vi "ep_Inverse Curves Constants.vi"(9 "other curves index":i32, 10 "IEEE curve type":u16(ring) items=["IEEE moderately inverse", "IEEE very inverse", "IEEE extremely inverse"], 11 "IEC curve type":u16(ring) items=["IEC inverse", "IEC very inverse", "IEC extremely inverse"]) -> (0 "other curve parameters":T1={"operate time parameters"={"A [s]"=1.0, "B [s]"=1.0, "alpha"=1.0, "K2 [s]"=1.0, "K1 [s]"=1.0, "K3 [s]"=1.0}, "reset time parameters"={"tr [s]"=1.0, "alpha"=1.0}}, 1 "difference of 1/time":fxp<+/-,21,-17>, 2 "1/time":fxp<+/-,30,-10>, 3 "number of sections in each G/Gs step":u16=8, 4 "IEC parameters":T1={"operate time parameters"={"A [s]"=1.0, "B [s]"=1.0, "alpha"=1.0, "K2 [s]"=1.0, "K1 [s]"=1.0, "K3 [s]"=1.0}, "reset time parameters"={"tr [s]"=1.0, "alpha"=1.0}}, 6 "IEEE parameters":T1={"operate time parameters"={"A [s]"=1.0, "B [s]"=1.0, "alpha"=1.0, "K2 [s]"=1.0, "K1 [s]"=1.0, "K3 [s]"=1.0}, "reset time parameters"={"tr [s]"=1.0, "alpha"=1.0}})   [LabVIEW 2012, in "NI_EP_Protection.lvlib"]
uses:
  <vilib>/addons/Electrical Power/Protection/NI_EP_Protection.lvlib
  <vilib>/addons/Electrical Power/Protection/Inverse Time Delay/subVIs/ep_Curve Parameters.ctl
  <vilib>/addons/Electrical Power/Protection/Inverse Time Delay/subVIs/ep_Operate Time.ctl
  <vilib>/addons/Electrical Power/Protection/Inverse Time Delay/subVIs/ep_Reset Time.ctl
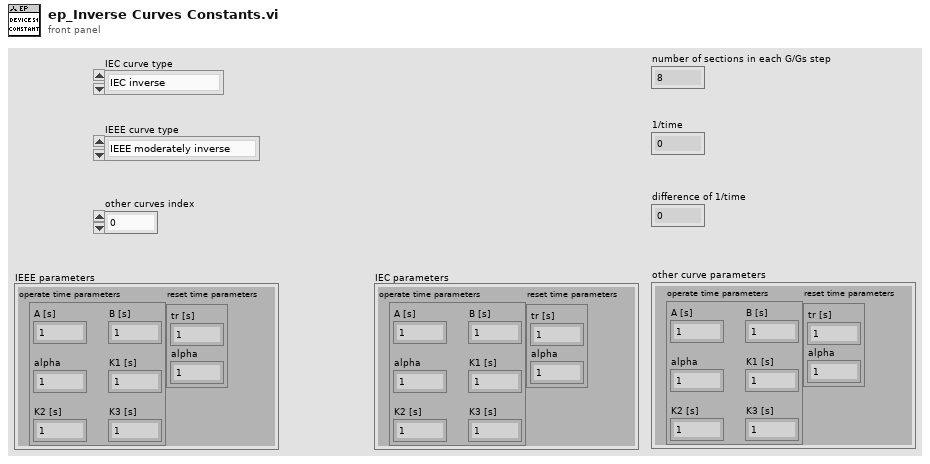
[diagram p1: front panel]
types:
  T1 = typedef "NI_EP_Protection.lvlib/ep_Curve Parameters.ctl" = cluster{"operate time parameters":T2, "reset time parameters":T3}
  T2 = typedef "NI_EP_Protection.lvlib/ep_Operate Time.ctl" = cluster{"A [s]":dbl, "B [s]":dbl, "alpha":dbl, "K2 [s]":dbl, "K1 [s]":dbl, "K3 [s]":dbl}
  T3 = typedef "NI_EP_Protection.lvlib/ep_Reset Time.ctl" = cluster{"tr [s]":dbl, "alpha":dbl}
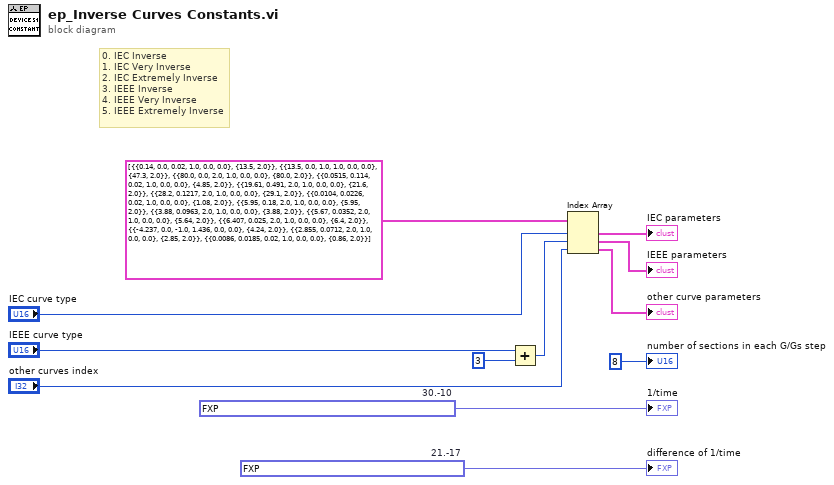
[diagram p0: block diagram]
diagram:
  w1 = fxp<+/-,21,-17> 3.814693627646193e-06  # 21.-17
  w2 = fxp<+/-,30,-10> 0.0004882812490905053  # 30.-10
  # "0. IEC Inverse\n1. IEC Very Inverse\n2. IEC Extremely Inverse\n3. IEEE Inverse\n4. IEEE Very Inverse\n5. IEEE Extremely Inverse"
  n1 = Add(x="IEEE curve type", y=3 ("index")) -> (x+y=w5:i32)
  n2 = Index Array(array=T1[] [{"operate time parameters"={"A [s]"=0.14, "B [s]"=0.0, "alpha"=0.02, "K2 [s]"=1.0, "K1 [s]"=0.0, "K3 [s]"=0.0}, "reset time parameters"={"tr [s]"=13.5, "alpha"=2.0}}, {"operate time parameters"={"A [s]"=13.5, "B [s]"=0.0, "alpha"=1.0, "K2 [s]"=1.0, "K1 [s]"=0.0, "K3 [s]"=0.0}, "reset time parameters"={"tr [s]"=47.3, "alpha"=2.0}}, {"operate time parameters"={"A [s]"=80.0, "B [s]"=0.0, "alpha"=2.0, "K2 [s]"=1.0, "K1 [s]"=0.0, "K3 [s]"=0.0}, "reset time parameters"={"tr [s]"=80.0, "alpha"=2.0}}, {"operate time parameters"={"A [s]"=0.0515, "B [s]"=0.114, "alpha"=0.02, "K2 [s]"=1.0, "K1 [s]"=0.0, "K3 [s]"=0.0}, "reset time parameters"={"tr [s]"=4.85, "alpha"=2.0}}, {"operate time parameters"={"A [s]"=19.61, "B [s]"=0.491, "alpha"=2.0, "K2 [s]"=1.0, "K1 [s]"=0.0, "K3 [s]"=0.0}, "reset time parameters"={"tr [s]"=21.6, "alpha"=2.0}}, {"operate time parameters"={"A [s]"=28.2, "B [s]"=0.1217, "alpha"=2.0, "K2 [s]"=1.0, "K1 [s]"=0.0, "K3 [s]"=0.0}, "reset time parameters"={"tr [s]"=29.1, "alpha"=2.0}}, {"operate time parameters"={"A [s]"=0.0104, "B [s]"=0.0226, "alpha"=0.02, "K2 [s]"=1.0, "K1 [s]"=0.0, "K3 [s]"=0.0}, "reset time parameters"={"tr [s]"=1.08, "alpha"=2.0}}, {"operate time parameters"={"A [s]"=5.95, "B [s]"=0.18, "alpha"=2.0, "K2 [s]"=1.0, "K1 [s]"=0.0, "K3 [s]"=0.0}, "reset time parameters"={"tr [s]"=5.95, "alpha"=2.0}}, {"operate time parameters"={"A [s]"=3.88, "B [s]"=0.0963, "alpha"=2.0, "K2 [s]"=1.0, "K1 [s]"=0.0, "K3 [s]"=0.0}, "reset time parameters"={"tr [s]"=3.88, "alpha"=2.0}}, {"operate time parameters"={"A [s]"=5.67, "B [s]"=0.0352, "alpha"=2.0, "K2 [s]"=1.0, "K1 [s]"=0.0, "K3 [s]"=0.0}, "reset time parameters"={"tr [s]"=5.64, "alpha"=2.0}}, {"operate time parameters"={"A [s]"=6.407, "B [s]"=0.025, "alpha"=2.0, "K2 [s]"=1.0, "K1 [s]"=0.0, "K3 [s]"=0.0}, "reset time parameters"={"tr [s]"=6.4, "alpha"=2.0}}, {"operate time parameters"={"A [s]"=-4.237, "B [s]"=0.0, "alpha"=-1.0, "K2 [s]"=1.436, "K1 [s]"=0.0, "K3 [s]"=0.0}, "reset time parameters"={"tr [s]"=4.24, "alpha"=2.0}}, {"operate time parameters"={"A [s]"=2.855, "B [s]"=0.0712, "alpha"=2.0, "K2 [s]"=1.0, "K1 [s]"=0.0, "K3 [s]"=0.0}, "reset time parameters"={"tr [s]"=2.85, "alpha"=2.0}}, {"operate time parameters"={"A [s]"=0.0086, "B [s]"=0.0185, "alpha"=0.02, "K2 [s]"=1.0, "K1 [s]"=0.0, "K3 [s]"=0.0}, "reset time parameters"={"tr [s]"=0.86, "alpha"=2.0}}] ("curve parameters"), index #1="IEC curve type", index #2=w5, index #3="other curves index") -> (element #1=→"IEC parameters":T1, element #2=→"IEEE parameters":T1, element #3=→"other curve parameters":T1)
  "number of sections in each G/Gs step" <- u16 8 ("number of sections in each G/Gs step")
  "1/time" <- w2
  "difference of 1/time" <- w1
